vi "FPGA_HoppingScan_BoostedMultiRegion.vi"() -> ()   [LabVIEW 2024]
uses:
  <vilib>/Platform/TimedLoop/XDataNode/timing_clust.ctl
  <vilib>/Platform/TimedLoop/XDataNode/nitl_modes.ctl
  <vilib>/Platform/TimedLoop/XDataNode/wakeup.ctl
  <vilib>/rvi/FXPMathLib/FxpDiv/subVIs/nifxpmath_Div_SimConfig.ctl
  <vilib>/rvi/Emulation/niFpgaSctlEmulationGetInTimedLoop.vi
  <vilib>/rvi/Emulation/niFpgaProcessEmulError.vi
  <vilib>/rvi/eio/common/nirviEmuTemplateMethod_errors.vi
  <vilib>/rvi/Memory/Memory_Emulation/nirvimemoryFastEmulation.vi
  <vilib>/rvi/Memory/Memory_Emulation/nirvimemoryEmulation.vi
  <vilib>/rvi/Emulation/niFpgaEmulationIsFPGAContextNoSignature.vi
  <vilib>/rvi/DataTransferAndStorage/Container/Common/niFpgaContainerGetUniqueNameForEmu.vi
  <vilib>/rvi/errors/nirviReportUnexpectedCaseInternalError (U32).vi
  <vilib>/rvi/Emulation/niFpgaEmulationReportErrorSimple.vi
  <vilib>/rvi/Emulation/niFpgaGetClockAttributes.vi
  <vilib>/rvi/Emulation/niFpgaCriticalErrorInLSC.vi
  <vilib>/rvi/Memory/Memory_Emulation/niFpgaMemoryEmulationCacheClearOnFirstRun.vi
  <vilib>/rvi/Memory/Memory_Emulation/nirvimemoryEmulationManagerCache_MakeExclusive.vi
  <vilib>/rvi/Memory/Memory_Emulation/niFpgaMemoryEmulationValidateCache.vi
  <vilib>/rvi/Memory/Memory_Emulation/nirvimemoryEmulationManagerCache_InsertValue.vi
  <vilib>/Utility/error.llb/Clear Errors.vi
  <vilib>/rvi/Memory/Memory_Emulation/nirvimemoryEmulationManagerCache_ReleaseExclusive.vi
  <vilib>/rvi/Memory/Memory_Emulation/nirvimemoryEmulationManagerCache_GetValue.vi
  <vilib>/rvi/Memory/Memory_Emulation/nirvimemoryEmulationManagerCache_SetValue.vi
  <vilib>/rvi/FIFO/Fifo_Resource/nirvififoEmulationSetSize.vi
  <vilib>/rvi/FIFO/Fifo_Resource/nirviFifoEmulationQueueMgr.vi
  <instcachedir>/0/nirviFifoEmulationQueueMgr_E5CAEC123FF24DC58D834DCA3CDAA9B5.lvgen/nirviFifoEmulationQueueMgr_E5CAEC123FF24DC58D834DCA3CDAA9B5_001.vi
  <vilib>/rvi/errors/niFpgaSetErrorForExecOnDevCompSimple.vi
  <vilib>/rvi/eio/common/nirviEmuReportErrorAndStop.vi
  <vilib>/rvi/FIFO/Fifo_Resource/nirvififoEmulationCreateLock.vi
  <vilib>/rvi/FIFO/Fifo_Resource/nirvififoEmulationObtainLock.vi
  <vilib>/rvi/FIFO/Fifo_Resource/nirvififoEmulationReleaseLock.vi
  <vilib>/rvi/occurrence/nirviWaitOnOccurrenceBase.vi
  <vilib>/rvi/errors/nirviReportUnexpectedCaseInternalError.vi
  <vilib>/eio/utilities/niEioResolveVilibRelativePath.vi
  <vilib>/rvi/interface/RandomDataEmulation/niFpgaRandomDataHandleErrors.vi
  <vilib>/rvi/FXPMathLib/FxpDiv/simVIs/DllFxpDivTemp_sub.vi
  <vilib>/rvi/FIFO/Fifo_Resource/nirvififoEmulationDetermineInputValidOut.vi
  <vilib>/eio/EIONode/EIONode.xnode
  <vilib>/rvi/DataTransferAndStorage/Container/XNode/niFpgaContainer.xnode
  <vilib>/platform/TimedLoop/XDataNode/XDataNode.xnode
  <vilib>/rvi/DataTransferAndStorage/Register/Emulation/niFpgaRegisterEmulation.vi
  <vilib>/rvi/FIFO/Fifo_Resource/nirvififoEmulationGetNumberOfElementsToRead.vi
  <vilib>/rvi/FIFO/Fifo_Resource/nirvififoEmulationRead.vi
  <vilib>/rvi/interface/RandomDataEmulation/nirviRandomDataFpgaReadWriteTemplate.vi
  <vilib>/rvi/FXPMathLib/FxpSub/XNode/nifxpmath_Sub.xnode
  <vilib>/rvi/FXPMathLib/FxpAdd/XNode/nifxpmath_Add.xnode
  <vilib>/rvi/FXPMathLib/FxpMul/XNode/nifxpmath_Multiplier.xnode
  <vilib>/rvi/FXPMathLib/FxpDiv/XNode/nifxpmath_Div.xnode
  <vilib>/rvi/FIFO/Fifo_Resource/nirvififoEmulationWrite.vi
  <vilib>/rvi/FXPMathLib/sim/FxpSim.dll
  <vilib>/Platform/TimedLoop/XDataNode/XDNodeRunTimeDep.lvlib
panel:
  in  "Turning Distance":fxp<+/-,48,16>
  in  "LastScan":bool
  in  "InitScan":bool
  in  "DelayPoints":i32
  in  "Halting Threshold":fxp<+/-,48,16>
  out "point_scanned":u32
  in  "TotalPoints":u32
  in  "RetRate us":i32
  in  "AppRate_NF us":i32
  in  "AppRate_FF us":i32
  in  "Recording Threshold":fxp<+/-,48,16>
  in  "stop":bool
  out "TargetDone?":bool
  out "ScanFinished?":bool
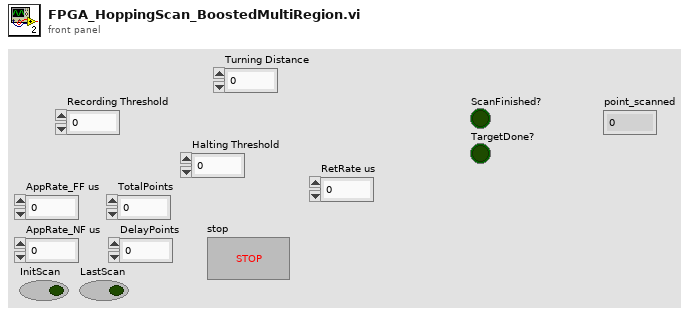
[diagram p1: front panel]
types:
  T1 = typedef "XDNodeRunTimeDep.lvlib/timing_clust.ctl" = cluster{"Expected End [f-1]":u64, "Actual End [f-1]":u64, "Finished Late? [f-1]":bool, "Expected End [i-1]":u64, "Actual End [i-1]":u64, "Finished Late? [i-1]":bool, "Expected Start [i]":u64, "Actual Start [i]":u64, "Expected Start [f]":u64, "Actual Start [f]":u64, "Source Name":string, "Structure Name":string, "Period":i64, "Deadline":i64, "Offset":i64, "Start":i64, "Priority":i32, "Timeout":i32, "Mode":T2, "Wakeup Reason":T3, "Error":errorcluster, "Source Type":string, "Secondary Source Type":string, "Global End Time":u64, "Global Start Time":u64, "Frame Duration":u64, "Iteration Duration":u64, "Assigned CPU":i32, "I/O Scan Engine Mode":u32}
  T2 = typedef "XDNodeRunTimeDep.lvlib/nitl_modes.ctl" = enum32{"No Change", "Process missed periods, maintain original phase", "Discard missed periods, maintain original phase", "Process missed periods, ignore original phase", "Discard missed periods, ignore original phase"}
  T3 = typedef "XDNodeRunTimeDep.lvlib/wakeup.ctl" = enum32{"Normal", "Aborted", "Asynchronous wakeup", "Timing source error", "Timed loop error", "Timeout"}
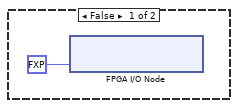
[diagram p2: hidden frame]
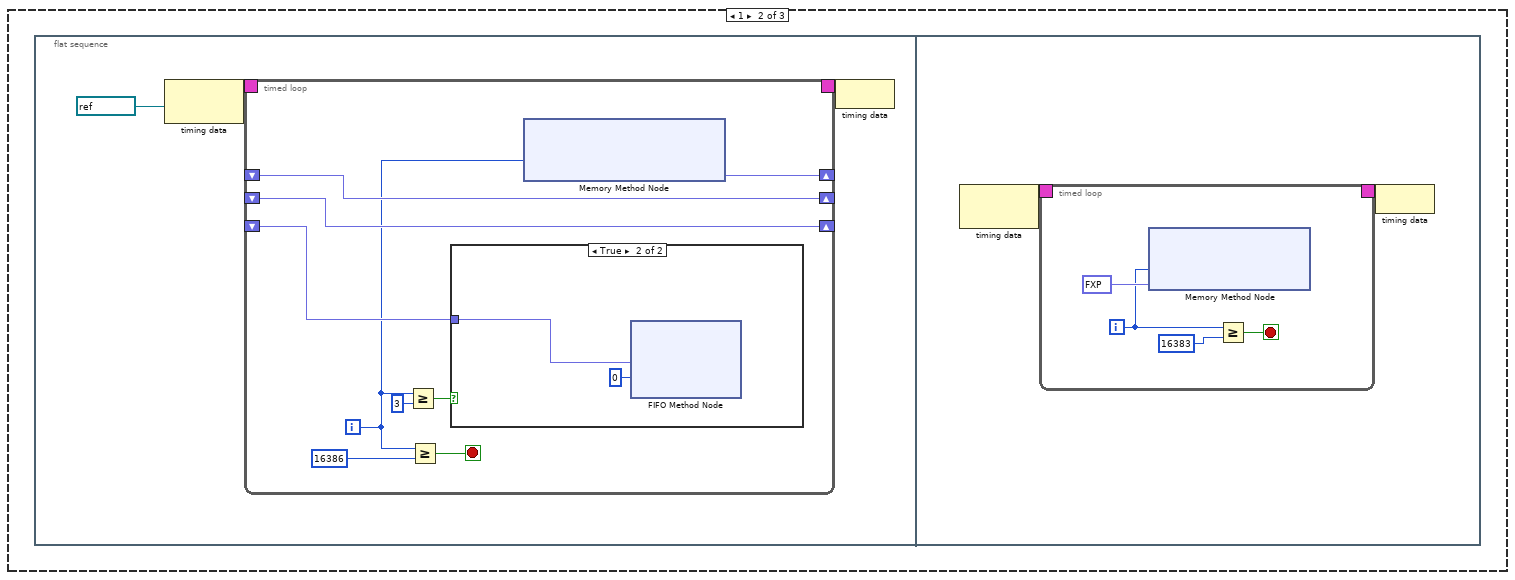
[diagram p5: hidden frame]
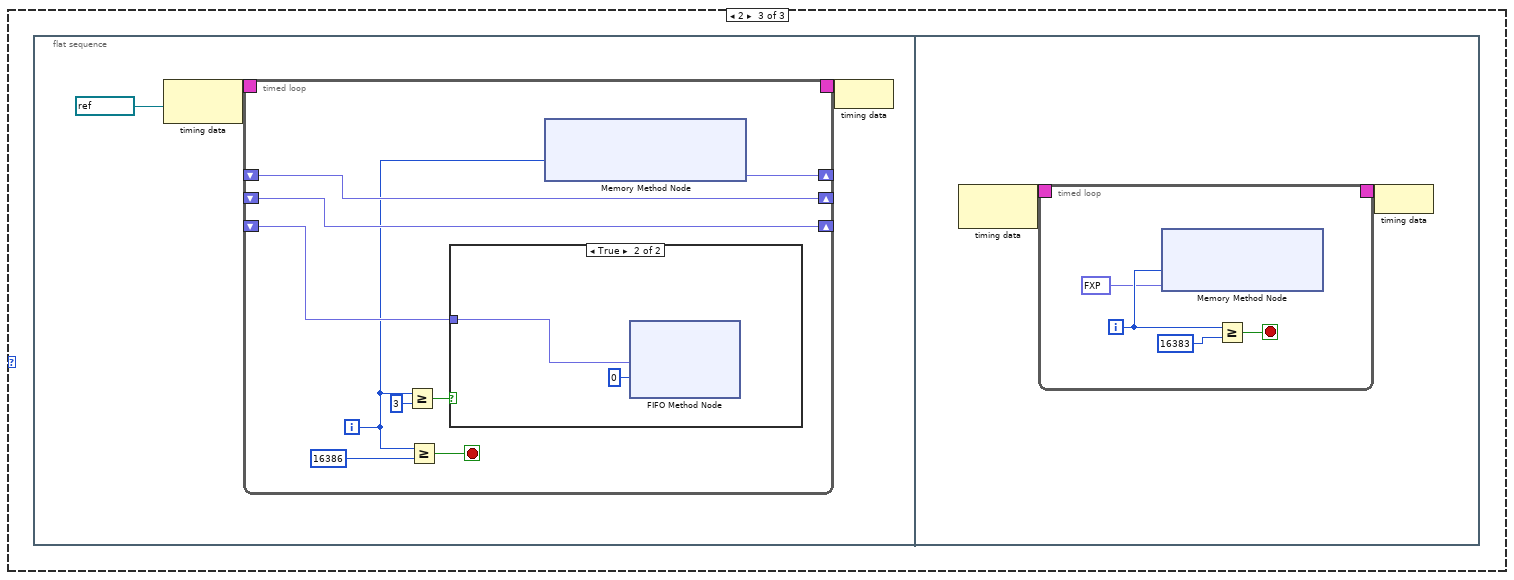
[diagram p7: hidden frame]
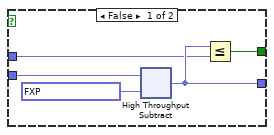
[diagram p14: hidden frame]
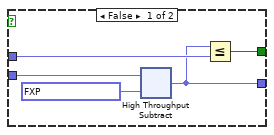
[diagram p15: hidden frame]
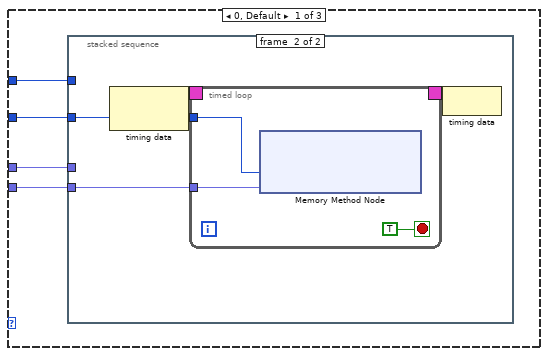
[diagram p18: hidden frame]
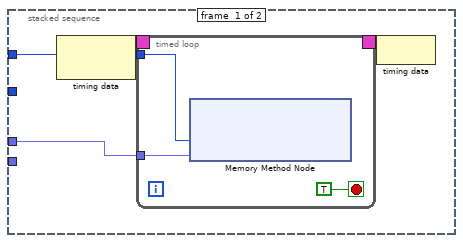
[diagram p19: hidden frame]
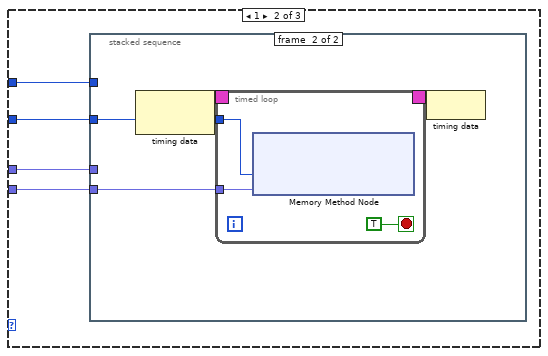
[diagram p20: hidden frame]
diagram:
  n1 = flat-sequence {
    tunnel: [w21] -> w1
    tunnel: w1 -> [w34]
    frame #0 {
      n2 = call "Wait18"("Count(mSec)"=u8 150) -> ()  [unwired: 1 out]
    }
    frame #1 {
      n3 = node-c288() -> (w5:T1)  [unwired: 1 in]
      n4 = timed-loop {
        timing: w5 -> [_]
        timing-out: [_] -> w4
        i -> [w14]
        stop <- w13 stop-if-true
        w16 = fxp<+/-,48,16> -100.0 ("Data")
        n5 = xnode ("Memory Method Node")("Address"=w14, "Data"=w16) -> ()  [unwired: 1 in, 1 out]
        n6 = xnode ("Memory Method Node")("Address"=w14, "Data"=w16) -> ()  [unwired: 1 in, 1 out]
        n7 = xnode ("Memory Method Node")("Address"=w14, "Data"=w16) -> ()  [unwired: 1 in, 1 out]
        n8 = Greater Or Equal?(x=w14, y=16383) -> (x >= y?=w13:bool)
      }
      n9 = case shown="True" "InitScan" {
        frame False {
          n10 = xnode "FPGA I/O Node"("Connector0/AO2"=fxp<+/-,20,5> 0.0 ("Connector0/AO0")) -> ()  [unwired: 1 in, 1 out]
        }
        frame True {
          w10 = fxp<+/-,20,5> 0.0 ("Connector0/AO0")
          n11 = for {
            N: 6 -> [_]
            i -> [w12]
            n12 = xnode ("Memory Method Node")("Address"=w12, "Data"=fxp<+/-,48,16> 0.0) -> ()  [unwired: 1 in, 1 out]
          }
          n13 = xnode "FPGA I/O Node"("Connector0/AO0"=w10, "Connector0/AO1"=w10, "Connector0/AO2"=w10) -> ()  [unwired: 3 in, 3 out]
        }
      }
      n14 = node-c288(w4) -> ()
      "ScanFinished?" <- FALSE
      "TargetDone?" <- FALSE
    }
    frame #2 {
      n15 = Generate Occurrence() -> (w21:refnum<k4>)
      n16 = call "Wait"("Count(mSec)"=u8 50) -> ()  [unwired: 1 out]
    }
    frame #3 {
      n17 = while {
        tunnel: w34 -> [w151]
        stop <- w153 stop-if-true
        n18 = xnode ("Register Read")() -> ("Data"=w154:bool)  [unwired: 1 in, 1 out]
        n19 = xnode ("FIFO Method Node")() -> ("Number of Elements to Read"=w157:u32)  [unwired: 1 in, 1 out]
        n20 = local read "ScanFinished?"() -> (w152:bool)
        n21 = Or(x=w154, y=w152) -> (x .or. y?=w153:bool)
        n22 = Greater Or Equal?(x=w157, y=u32 6) -> (x >= y?=w155:bool)
        n23 = case shown="True" w155 {
          tunnel: w151 -> [_ w158]
          frame False {
          }
          frame True {
            n24 = First Call?() -> (First Call?: T/F=w159:bool)
            n25 = case shown="True" w159 {
              tunnel: w158 -> [_ w160]
              frame False {
              }
              frame True {
                n26 = flat-sequence {
                  tunnel: [w163] -> w161
                  tunnel: w160 -> [w163]
                  tunnel: w161 -> [w164]
                  frame #0 {
                    n27 = call "Wait3"("Count(mSec)"=u8 4) -> ()  [unwired: 1 out]
                  }
                  frame #1 {
                    n28 = Set Occurrence(w164) -> ()
                  }
                }
              }
            }
          }
        }
      }
      n29 = while {
        tunnel: w34 -> [w136]
        stop <- w133 stop-if-true
        n30 = flat-sequence {
          tunnel: ["stop"] -> w138
          tunnel: w136 -> [w140]
          tunnel: [w140] -> w134
          tunnel: w138 -> [w143]
          tunnel: [w143] -> w137
          tunnel: [w142] -> w135
          tunnel: w134 -> [w142]
          tunnel: w137 -> [w147]
          tunnel: w135 -> [w146]
          tunnel: [w145] -> w133
          frame #0 {
            n31 = case shown="True" "stop" {
              tunnel: "stop" -> [_ w141]
              frame False {
              }
              frame True {
                n32 = xnode ("Register Write")("Data"=w141) -> ()  [unwired: 1 in, 1 out]
              }
            }
          }
          frame #1 {
            n33 = call "Wait2"("Count(uSec)"=u8 200) -> ()  [unwired: 1 out]
          }
          frame #2 {
            n34 = xnode ("Register Read")() -> ("Data"=w148:bool)  [unwired: 1 in, 1 out]
            n35 = local read "ScanFinished?"() -> (w149:bool)
            n36 = Compound Arithmetic op=OR(w149, w148, w147) -> (w145:bool)
            n37 = case shown="True" w145 {
              tunnel: w146 -> [_ w150]
              frame False {
              }
              frame True {
                n38 = Set Occurrence(w150) -> ()
              }
            }
          }
        }
      }
      n39 = flat-sequence {
        tunnel: w34 -> [w165]
        tunnel: [fxp<+/-,48,16> 0.0 ("Threshold")] -> w33
        tunnel: [w167] -> w31
        tunnel: [u8 0] -> w28
        tunnel: w33 -> [w170]
        tunnel: [w171] -> w32
        tunnel: w31 -> [w171]
        tunnel: [w170] -> w30
        tunnel: [w169] -> w29
        tunnel: w28 -> [w169]
        tunnel: w32 -> [w176]
        tunnel: w30 -> [w175]
        tunnel: w29 -> [w174]
        tunnel: [w173] -> w27
        tunnel: w27 -> [w1243]
        tunnel: [w1242] -> w26
        tunnel: [w1241] -> w24
        tunnel: w26 -> [w1255]
        tunnel: [w1255] -> w25
        tunnel: w24 -> [w1254]
        tunnel: [w1254] -> w23
        tunnel: w25 -> [w1260]
        tunnel: w23 -> [w1259]
        frame #0 {
          n40 = Wait on Occurrence(2:w165) -> ()  [unwired: 2 in, 1 out]
        }
        frame #1 {
          # "z piezo voltage"
          # "Swapchain indicator"
          n41 = xnode ("Register Read")() -> ("Data"=w167:bool)  [unwired: 1 in, 1 out]
        }
        frame #2 {
          n42 = call "Wait4"("Count(mSec)"=u8 4) -> ()  [unwired: 1 out]
        }
        frame #3 {
          n43 = case shown="False" w176 {
            tunnel: w175 -> [w179 w1239]
            tunnel: w174 -> [w178 _]
            tunnel: [w177 w1239] -> w173
            frame False {
              n44 = while {
                shift-right: [w186] -> w177
                shift-left: w179 -> [w213]
                shift-right: [w185] -> _
                shift-left: w178 -> [w196]
                stop <- w184 stop-if-true
                n45 = flat-sequence {
                  tunnel: w213 -> [w215]
                  tunnel: [w217] -> w212
                  tunnel: [w216] -> w208
                  tunnel: [w215] -> w200
                  tunnel: w196 -> [w214]
                  tunnel: [w214] -> w195
                  tunnel: w212 -> [w225]
                  tunnel: [w225] -> w211
                  tunnel: w208 -> [w224]
                  tunnel: [w224] -> w207
                  tunnel: w200 -> [w223]
                  tunnel: [w223] -> w199
                  tunnel: w195 -> [w222]
                  tunnel: [w222] -> w194
                  tunnel: w211 -> [w252]
                  tunnel: [w252] -> w210
                  tunnel: [w245] -> w209
                  tunnel: w207 -> [w251]
                  tunnel: [w251] -> w206
                  tunnel: [w246] -> w205
                  tunnel: [w249] -> w204
                  tunnel: [w248] -> w203
                  tunnel: [w247] -> w202
                  tunnel: w199 -> [w244]
                  tunnel: w194 -> [w250]
                  tunnel: [w250] -> w193
                  tunnel: [w241] -> w183
                  tunnel: [w243] -> w180
                  tunnel: [w289] -> w201
                  tunnel: [w288] -> w198
                  tunnel: [w287] -> w191
                  tunnel: [w286] -> w190
                  tunnel: [w285] -> w189
                  tunnel: [w284] -> w182
                  tunnel: w180 -> [w288]
                  tunnel: w183 -> [w284]
                  tunnel: w193 -> [w287]
                  tunnel: w202 -> [w285]
                  tunnel: w203 -> [w286]
                  tunnel: w204 -> [w289]
                  tunnel: w205 -> [w291]
                  tunnel: w206 -> [w290]
                  tunnel: w209 -> [w281]
                  tunnel: w210 -> [w280]
                  tunnel: w201 -> [w335]
                  tunnel: w198 -> [w334]
                  tunnel: [w334] -> w197
                  tunnel: [w333] -> w192
                  tunnel: w191 -> [w333]
                  tunnel: w190 -> [w332]
                  tunnel: w189 -> [w331]
                  tunnel: [w332] -> w188
                  tunnel: [w331] -> w187
                  tunnel: w182 -> [w330]
                  tunnel: [w330] -> w181
                  tunnel: w197 -> [w350]
                  tunnel: w192 -> [w349]
                  tunnel: w188 -> [w348]
                  tunnel: w187 -> [w347]
                  tunnel: [w346] -> w185
                  tunnel: [w345] -> w186
                  tunnel: [w344] -> w184
                  tunnel: w181 -> [w340]
                  frame #0 {
                    # "Data from target to host:\n0, 1: X, Y piezo voltage\n2, 3: X, Y piezo idx\n4: Z piezo probing voltage\n5: Z piezo final voltage\n6: baseline current\n7: circular buffer pointer idx\n(8-8107): Z voltage\n(8108-16207): current\n(8107-16206): current"
                    # "Data from host to target:\n0, 1: X, Y piezo voltage\n2, 3: X, Y piezo idx\n4: distance (piezo voltage) to the last point\n5: retract height, \nall negative cases won't trigger approach of z piezo\nif -20, keep z and move xy\nif -30, full retract for z and move xy"
                    n46 = for {
                      N: 2 -> [_]
                      shift-right: [w221] -> w216
                      shift-left: _ -> [w219]
                      shift-right: [w219] -> w217
                      shift-left: _ -> [_]
                      i -> [w220]
                      n47 = xnode ("Memory Method Node")("Address"=w220) -> ("Data"=w221:fxp<+/-,48,16>)  [unwired: 1 in, 1 out]
                    }
                  }
                  frame #1 {
                    # "y"
                    # "x"
                    n48 = while {
                      shift-right: [w229] -> _
                      shift-left: i16 0 -> [w228]
                      stop <- w230 stop-if-true
                      n49 = xnode ("FIFO Method Node")("Timeout"=8192) -> ("Element"=w227:fxp<+/-,48,16>, "Timed Out?"=w234:bool)  [unwired: 1 in, 1 out]
                      n50 = Increment(x=w228) -> (x+1=w237:i16)
                      n51 = xnode ("Register Read")() -> ("Data"=w231:bool)  [unwired: 1 in, 1 out]
                      n52 = Select(t=w228, s=w234, f=w237) -> (s? t:f=w229:i16)
                      n53 = Not(x=w234) -> (.not. x?=w233:bool)
                      n54 = Equal?(x=w228, y=i16 5) -> (x = y?=w235:bool)
                      n55 = And(x=w235, y=w233) -> (x .and. y?=w232:bool)
                      n56 = xnode ("Memory Method Node")("Address"=w228, "Data"=w227) -> ()  [unwired: 1 in, 1 out]
                      n57 = Or(x=w232, y=w231) -> (x .or. y?=w230:bool)
                    }
                  }
                  frame #2 {
                    # "0"
                    # "5"
                    n58 = for {
                      N: 6 -> [_]
                      shift-right: [w278] -> w241
                      shift-left: _ -> [w277]
                      shift-right: [w277] -> w249
                      shift-left: _ -> [w276]
                      shift-right: [w276] -> w248
                      shift-left: _ -> [w275]
                      shift-right: [w275] -> w247
                      shift-left: _ -> [w274]
                      shift-right: [w274] -> w246
                      shift-left: _ -> [w273]
                      shift-right: [w273] -> w245
                      shift-left: _ -> [_]
                      i -> [w279]
                      n59 = xnode ("Memory Method Node")("Address"=w279) -> ("Data"=w278:fxp<+/-,48,16>)  [unwired: 1 in, 1 out]
                    }
                    n60 = Equal?(x=w241, y=fxp<+/-,48,16> -30.0) -> (x = y?=w240:bool)
                    n61 = case shown="True" w240 {
                      tunnel: w244 -> [w254 w258]
                      tunnel: [w254 w257] -> w243
                      tunnel: fxp<+/-,48,16> 0.0048828125 ("y") -> [_ w256]
                      frame False {
                      }
                      frame True {
                        n62 = flat-sequence {
                          tunnel: w258 -> [w261]
                          tunnel: w256 -> [w259]
                          tunnel: [w260] -> w255
                          tunnel: [w272] -> w257
                          tunnel: w255 -> [w272]
                          frame #0 {
                            n63 = while {
                              shift-right: [w265] -> w260
                              shift-left: w261 -> [w270]
                              tunnel: w259 -> [w264]
                              stop <- w266 stop-if-true
                              w267 = fxp<+/-,48,16> 0.0 ("y")
                              n64 = xnode "High Throughput Subtract"("x"=w270, "y"=w264) -> ("x-y"=w268:fxp<+/-,48,16>)
                              n65 = xnode ("Register Read")() -> ("Data"=w269:bool)  [unwired: 1 in, 1 out]
                              n66 = Less Or Equal?(x=w268, y=w267) -> (x <= y?=w262:bool)
                              n67 = Select(t=w267, s=w262, f=w268) -> (s? t:f=w265:fxp<+/-,48,16>)
                              n68 = local read "RetRate us"() -> (w263:i32)
                              n69 = xnode "FPGA I/O Node"("Connector0/AO2"=w265) -> ()  [unwired: 1 in, 1 out]
                              n70 = Compound Arithmetic op=OR(w262, w269) -> (w266:bool)
                              n71 = call "Wait10"("Count(uSec)"=w263) -> ()  [unwired: 1 out]
                            }
                          }
                          frame #1 {
                            n72 = call "Wait17"("Count(mSec)"=u16 2 ("Count(uSec)")) -> ()  [unwired: 1 out]
                          }
                        }
                      }
                    }
                  }
                  frame #3 {
                    n73 = xnode "High Throughput Subtract"("x"=w290, "y"=w291) -> ("x-y"=w293:fxp<+/-,48,16>)
                    n74 = xnode "High Throughput Subtract"("x"=w280, "y"=w281) -> ("x-y"=w283:fxp<+/-,48,16>)
                    n75 = Less Or Equal To 0?(x=w293) -> (x <= 0?=w292:bool)
                    n76 = Less Or Equal To 0?(x=w283) -> (x <= 0?=w282:bool)
                    n77 = while {
                      tunnel: w292 -> [w319]
                      tunnel: w291 -> [w318]
                      shift-right: [w312] -> _
                      shift-left: w290 -> [w314]
                      stop <- w315 stop-if-true
                      n78 = case shown="True" w319 {
                        tunnel: w318 -> [w321 w326]
                        tunnel: w314 -> [w323 w329]
                        tunnel: [w322 w327] -> w313
                        tunnel: [w320 w325] -> w312
                        frame False {
                          n79 = xnode "High Throughput Subtract"("x"=w323, "y"=fxp<+/-,48,16> 0.00030517578125) -> ("x-y"=w320:fxp<+/-,48,16>)
                          n80 = Less Or Equal?(x=w320, y=w321) -> (x <= y?=w322:bool)
                        }
                        frame True {
                          n81 = xnode ("High Throughput Add")("x"=w329, "y"=fxp<+/-,48,16> 0.00030517578125) -> ("x+y"=w325:fxp<+/-,48,16>)
                          n82 = Greater Or Equal?(x=w325, y=w326) -> (x >= y?=w327:bool)
                        }
                      }
                      n83 = call "Wait6"("Count(uSec)"=u32 70) -> ()  [unwired: 1 out]
                      n84 = xnode ("Register Read")() -> ("Data"=w316:bool)  [unwired: 1 in, 1 out]
                      n85 = xnode "FPGA I/O Node"("Connector0/AO1"=w312) -> ()  [unwired: 1 in, 1 out]
                      n86 = Or(x=w313, y=w316) -> (x .or. y?=w315:bool)
                    }
                    n87 = while {
                      tunnel: w282 -> [w301]
                      tunnel: w281 -> [w300]
                      shift-right: [w294] -> _
                      shift-left: w280 -> [w296]
                      stop <- w297 stop-if-true
                      n88 = case shown="True" w301 {
                        tunnel: w300 -> [w302 w307]
                        tunnel: w296 -> [w305 w311]
                        tunnel: [w304 w309] -> w295
                        tunnel: [w303 w308] -> w294
                        frame False {
                          n89 = xnode "High Throughput Subtract"("x"=w305, "y"=fxp<+/-,48,16> 0.00030517578125) -> ("x-y"=w303:fxp<+/-,48,16>)
                          n90 = Less Or Equal?(x=w303, y=w302) -> (x <= y?=w304:bool)
                        }
                        frame True {
                          n91 = xnode ("High Throughput Add")("x"=w311, "y"=fxp<+/-,48,16> 0.00030517578125) -> ("x+y"=w308:fxp<+/-,48,16>)
                          n92 = Greater Or Equal?(x=w308, y=w307) -> (x >= y?=w309:bool)
                        }
                      }
                      n93 = call "Wait5"("Count(uSec)"=u32 70) -> ()  [unwired: 1 out]
                      n94 = xnode ("Register Read")() -> ("Data"=w298:bool)  [unwired: 1 in, 1 out]
                      n95 = xnode "FPGA I/O Node"("Connector0/AO0"=w294) -> ()  [unwired: 1 in, 1 out]
                      n96 = Or(x=w295, y=w298) -> (x .or. y?=w297:bool)
                    }
                  }
                  frame #4 {
                    n97 = xnode ("High Throughput Multiply")("x"=w335, "y"=fxp<+/-,48,16> 1600.0) -> ("x*y"=w337:fxp<+/-,52,20>)
                    n98 = To Unsigned Long Integer(number=w337) -> (unsigned 32bit integer=w338:u32)
                    n99 = call "Wait7"("Count(uSec)"=w338) -> ()  [unwired: 1 out]
                  }
                  frame #5 {
                    # "Y, X idx"
                    n100 = xnode ("Register Read")() -> ("Data"=w343:bool)  [unwired: 1 in, 1 out]
                    n101 = Less Or Equal?(x=w340, y=fxp<+/-,48,16> -20.0) -> (x <= y?=w341:bool)
                    n102 = Or(x=w341, y=w343) -> (x .or. y?=w342:bool)
                    n103 = case shown="False" w342 {
                      tunnel: w350 -> [w397 w1238]
                      tunnel: w349 -> [w396 w1237]
                      tunnel: w348 -> [w392 _]
                      tunnel: w347 -> [w391 _]
                      tunnel: [w389 w1238] -> w345
                      tunnel: [w390 w1237] -> w346
                      tunnel: [w388 w1234] -> w344
                      tunnel: w341 -> [_ w1236]
                      tunnel: w340 -> [w384 _]
                      frame False {
                        n104 = flat-sequence {
                          tunnel: [w399] -> w382
                          tunnel: [w404] -> w381
                          tunnel: [w403] -> w380
                          tunnel: w397 -> [w402]
                          tunnel: [w402] -> w379
                          tunnel: w396 -> [w401]
                          tunnel: [w401] -> w378
                          tunnel: [0] -> w377
                          tunnel: [w399] -> w376
                          tunnel: w382 -> [w442]
                          tunnel: [w441] -> w375
                          tunnel: w381 -> [w443]
                          tunnel: w380 -> [w449]
                          tunnel: [w449] -> w374
                          tunnel: w379 -> [w445]
                          tunnel: [w444] -> w373
                          tunnel: w378 -> [w448]
                          tunnel: [w448] -> w372
                          tunnel: w377 -> [w447]
                          tunnel: [w447] -> w371
                          tunnel: w376 -> [w446]
                          tunnel: [w446] -> w370
                          tunnel: [w440] -> w369
                          tunnel: w375 -> [w533]
                          tunnel: [w533] -> w364
                          tunnel: w374 -> [w532]
                          tunnel: [w532] -> w362
                          tunnel: w373 -> [w524]
                          tunnel: [w522] -> w360
                          tunnel: w372 -> [w531]
                          tunnel: [w531] -> w358
                          tunnel: w371 -> [w530]
                          tunnel: [w530] -> w356
                          tunnel: w370 -> [w529]
                          tunnel: [w529] -> w354
                          tunnel: w369 -> [w521]
                          tunnel: [w521] -> w352
                          tunnel: w364 -> [w558]
                          tunnel: [w558] -> w363
                          tunnel: w362 -> [w557]
                          tunnel: [w557] -> w361
                          tunnel: w360 -> [w556]
                          tunnel: [w556] -> w359
                          tunnel: w358 -> [w555]
                          tunnel: [w555] -> w357
                          tunnel: w356 -> [w554]
                          tunnel: [w554] -> w355
                          tunnel: w354 -> [w553]
                          tunnel: [w553] -> w353
                          tunnel: w352 -> [w552]
                          tunnel: [w552] -> w351
                          tunnel: w363 -> [w568]
                          tunnel: w361 -> [w567]
                          tunnel: w359 -> [w566]
                          tunnel: w357 -> [w565]
                          tunnel: w355 -> [w560]
                          tunnel: [w564] -> w395
                          tunnel: [w563] -> w394
                          tunnel: [w562] -> w393
                          tunnel: w353 -> [w561]
                          tunnel: [w561] -> w383
                          tunnel: w351 -> [w559]
                          tunnel: [w559] -> w368
                          tunnel: w395 -> [w851]
                          tunnel: w394 -> [w853]
                          tunnel: w393 -> [w854]
                          tunnel: w392 -> [w856]
                          tunnel: w391 -> [w855]
                          tunnel: [w852] -> w387
                          tunnel: [w851] -> w386
                          tunnel: [w848] -> w385
                          tunnel: w383 -> [w847]
                          tunnel: w368 -> [w846]
                          tunnel: w387 -> [w1211]
                          tunnel: w386 -> [w1207]
                          tunnel: w385 -> [w1210]
                          tunnel: w384 -> [w1208]
                          tunnel: [w1211] -> w367
                          tunnel: [w1209] -> w366
                          tunnel: [w1210] -> w365
                          tunnel: [w1230] -> w388
                          tunnel: [w1231] -> w389
                          tunnel: [w1232] -> w390
                          tunnel: w367 -> [w1232]
                          tunnel: w366 -> [w1231]
                          tunnel: w365 -> [w1230]
                          frame #0 {
                            n105 = for {
                              N: 32 -> [_]
                              shift-right: [w437] -> w407
                              shift-left: fxp<+/-,48,16> 0.0 -> [w438]
                              n106 = xnode "FPGA I/O Node"() -> ("Connector0/AI3"=w439:fxp<+/-,27,5>)  [unwired: 1 in, 1 out]
                              n107 = xnode ("High Throughput Add")("x"=w439, "y"=w438) -> ("x+y"=w437:fxp<+/-,48,16>)
                            }
                            n108 = local read "Halting Threshold"() -> (w398:fxp<+/-,48,16>)
                            n109 = local read "Recording Threshold"() -> (w405:fxp<+/-,48,16>)
                            n110 = xnode "High Throughput Divide"("x"=w407, "y"=fxp<+/-,48,16> 32.0) -> ("x/y"=w399:fxp<+/-,48,16>)
                            n111 = xnode ("High Throughput Multiply")("x"=w399, "y"=w405) -> ("x*y"=w404:fxp<+/-,48,16>)
                            n112 = xnode ("High Throughput Multiply")("x"=w399, "y"=w398) -> ("x*y"=w403:fxp<+/-,48,16>)
                          }
                          frame #1 {
                            n113 = while {
                              shift-right: [w451] -> w444
                              shift-left: w445 -> [w457]
                              tunnel: w443 -> [w462]
                              tunnel: w442 -> [w461]
                              tunnel: [w460] -> w441
                              tunnel: [w450] -> w440
                              stop <- w454 stop-if-true
                              n114 = flat-sequence {
                                tunnel: w462 -> [w475]
                                tunnel: w461 -> [w477]
                                tunnel: [w477] -> w459
                                tunnel: w457 -> [w464]
                                tunnel: [w466] -> w455
                                tunnel: [w463] -> w453
                                tunnel: w459 -> [w516]
                                tunnel: [w516] -> w458
                                tunnel: [w515] -> w456
                                tunnel: w455 -> [w515]
                                tunnel: w453 -> [w514]
                                tunnel: [w514] -> w452
                                tunnel: [w520] -> w460
                                tunnel: w458 -> [w520]
                                tunnel: w456 -> [w519]
                                tunnel: [w519] -> w454
                                tunnel: w452 -> [w517]
                                tunnel: [w517] -> w451
                                tunnel: [w517] -> w450
                                frame #0 {
                                w483 = 16
                                n115 = for {
                                N: w483 -> [_]
                                shift-right: [w511] -> w481
                                shift-left: fxp<+/-,48,16> 0.0 ("y") -> [w513]
                                n116 = xnode "FPGA I/O Node"() -> ("Connector0/AI3"=w512:fxp<+/-,27,5>)  [unwired: 2 in, 3 out]
                                n117 = xnode ("High Throughput Add")("x"=w513, "y"=w512) -> ("x+y"=w511:fxp<+/-,48,16>)
                                }
                                n118 = To Fixed-Point(number=w483) -> (fixed-point=w482:fxp<+/-,48,16>)  [unwired: 1 in]
                                n119 = xnode ("High Throughput Add")("x"=w464, "y"=fxp<+/-,48,16> 0.00030517578125) -> ("x+y"=w465:fxp<+/-,48,16>)
                                n120 = xnode ("Register Read")() -> ("Data"=w467:bool)  [unwired: 1 in, 1 out]
                                n121 = Greater?(x=w465, y=fxp<+/-,48,16> 9.75) -> (0:w473:bool)
                                n122 = Less?(x=w465, y=fxp<+/-,48,16> -0.125) -> (x < y?=w474:bool)
                                n123 = Or(x=w474, y=w473) -> (x .or. y?=w468:bool)
                                n124 = xnode "High Throughput Divide"("x"=w481, "y"=w482) -> ("x/y"=w478:fxp<+/-,48,16>)
                                n125 = xnode "High Throughput Subtract"("x"=w477, "y"=w478) -> ("x-y"=w479:fxp<+/-,48,16>)
                                n126 = Absolute Value(x=w479) -> (abs(x)=w476:fxp<+,48,16>)
                                n127 = Greater Or Equal?(x=w476, y=w475) -> (x >= y?=w469:bool)
                                n128 = Compound Arithmetic op=OR(w469, w467, w468) -> (w466:bool)
                                n129 = Select(t=w464, s=w466, f=w465) -> (s? t:f=w463:fxp<+/-,48,16>)
                                }
                                frame #1 {
                                n130 = xnode "FPGA I/O Node"("Connector0/AO2"=w514) -> ()  [unwired: 1 in, 1 out]
                                }
                                frame #2 {
                                n131 = local read "AppRate_FF us"() -> (w518:i32)
                                n132 = call "Wait19"("Count(uSec)"=w518) -> ()  [unwired: 1 out]
                                }
                              }
                            }
                          }
                          frame #2 {
                            n133 = xnode ("Register Read")() -> ("Data"=w528:bool)  [unwired: 1 in, 1 out]
                            n134 = local read "Turning Distance"() -> (w523:fxp<+/-,48,16>)
                            n135 = Less Or Equal To 0?(x=w524) -> (x <= 0?=w527:bool)
                            n136 = Or(x=w528, y=w527) -> (x .or. y?=w526:bool)
                            n137 = case shown="False" w526 {
                              tunnel: w524 -> [w536 w550]
                              tunnel: [w538 w550] -> w522
                              tunnel: fxp<+/-,48,16> 0.00030517578125 ("y") -> [w537 _]
                              tunnel: w523 -> [w534 _]
                              frame False {
                                n138 = xnode "High Throughput Subtract"("x"=w536, "y"=w534) -> ("x-y"=w535:fxp<+/-,48,16>)
                                n139 = while {
                                shift-right: [w543] -> w538
                                shift-left: w536 -> [w549]
                                tunnel: w537 -> [w542]
                                tunnel: w535 -> [w541]
                                stop <- w544 stop-if-true
                                n140 = xnode "High Throughput Subtract"("x"=w549, "y"=w542) -> ("x-y"=w545:fxp<+/-,48,16>)
                                n141 = xnode ("Register Read")() -> ("Data"=w548:bool)  [unwired: 1 in, 1 out]
                                n142 = Less Or Equal To 0?(x=w545) -> (x <= 0?=w546:bool)
                                n143 = Less Or Equal?(x=w545, y=w541) -> (x <= y?=w547:bool)
                                n144 = Select(t=fxp<+/-,48,16> 0.0, s=w546, f=w545) -> (s? t:f=w543:fxp<+/-,48,16>)
                                n145 = local read "RetRate us"() -> (w539:i32)
                                n146 = xnode "FPGA I/O Node"("Connector0/AO2"=w543) -> ()  [unwired: 1 in, 1 out]
                                n147 = Compound Arithmetic op=OR(w546, w547, w548) -> (w544:bool)
                                n148 = call "Wait20"("Count(uSec)"=w539) -> ()  [unwired: 1 out]
                                }
                              }
                              frame True {
                              }
                            }
                          }
                          frame #3 {
                            n149 = call "Wait22"("Count(mSec)"=u8 5) -> ()  [unwired: 1 out]
                          }
                          frame #4 {
                            n150 = while {
                              tunnel: w568 -> [w614]
                              tunnel: w567 -> [w613]
                              shift-right: [w597] -> w564
                              shift-left: w566 -> [w612]
                              shift-right: [w596] -> w563
                              shift-left: w565 -> [w611]
                              shift-right: [w582] -> _
                              shift-left: w560 -> [w604]
                              tunnel: [w590] -> w562
                              shift-right: [w569] -> _
                              shift-left: w560 -> [w573]
                              stop <- w593 stop-if-true
                              n151 = flat-sequence {
                                tunnel: w604 -> [w617]
                                tunnel: w611 -> [w618]
                                tunnel: w612 -> [w619]
                                tunnel: w613 -> [w620]
                                tunnel: w614 -> [w621]
                                tunnel: [w621] -> w589
                                tunnel: [w620] -> w588
                                tunnel: [w619] -> w587
                                tunnel: [w618] -> w586
                                tunnel: [w617] -> w585
                                tunnel: [w616] -> w584
                                tunnel: [w615] -> w574
                                tunnel: w573 -> [w615]
                                tunnel: [w655] -> w610
                                tunnel: [w643] -> w608
                                tunnel: [w640] -> w607
                                tunnel: [w654] -> w603
                                tunnel: [w653] -> w601
                                tunnel: [w652] -> w598
                                tunnel: [w635] -> w595
                                tunnel: [w645] -> w591
                                tunnel: w589 -> [w659]
                                tunnel: w588 -> [w636]
                                tunnel: w587 -> [w656]
                                tunnel: w586 -> [w653]
                                tunnel: w585 -> [w654]
                                tunnel: w584 -> [w639]
                                tunnel: [w639] -> w583
                                tunnel: w574 -> [w627]
                                tunnel: [w628] -> w571
                                tunnel: w610 -> [w729]
                                tunnel: [w729] -> w609
                                tunnel: w608 -> [w728]
                                tunnel: w607 -> [w727]
                                tunnel: [w728] -> w606
                                tunnel: [w727] -> w605
                                tunnel: w603 -> [w726]
                                tunnel: [w726] -> w602
                                tunnel: w601 -> [w725]
                                tunnel: [w725] -> w600
                                tunnel: [w724] -> w599
                                tunnel: w598 -> [w724]
                                tunnel: w595 -> [w723]
                                tunnel: [w723] -> w594
                                tunnel: [w722] -> w592
                                tunnel: w591 -> [w722]
                                tunnel: w583 -> [w721]
                                tunnel: [w721] -> w576
                                tunnel: [w720] -> w572
                                tunnel: w571 -> [w720]
                                tunnel: w609 -> [w741]
                                tunnel: w606 -> [w743]
                                tunnel: w605 -> [w742]
                                tunnel: w602 -> [w732]
                                tunnel: w600 -> [w740]
                                tunnel: w599 -> [w734]
                                tunnel: w594 -> [w739]
                                tunnel: w592 -> [w738]
                                tunnel: [w744] -> w581
                                tunnel: [w741] -> w580
                                tunnel: [w740] -> w579
                                tunnel: [w739] -> w578
                                tunnel: [w738] -> w577
                                tunnel: w576 -> [w736]
                                tunnel: [w736] -> w575
                                tunnel: w572 -> [w735]
                                tunnel: [w735] -> w570
                                tunnel: [w841] -> w590
                                tunnel: [w842] -> w593
                                tunnel: [w843] -> w596
                                tunnel: [w844] -> w597
                                tunnel: [w845] -> w582
                                tunnel: w581 -> [w845]
                                tunnel: w580 -> [w844]
                                tunnel: w579 -> [w843]
                                tunnel: w578 -> [w842]
                                tunnel: w577 -> [w841]
                                tunnel: w575 -> [w839]
                                tunnel: [w833] -> w569
                                tunnel: w570 -> [w833]
                                frame #0 {
                                n152 = call "Tick Count"() -> ("Tick Count(uSec)"=w616:u32)
                                }
                                frame #1 {
                                w625 = 16
                                w657 = fxp<+/-,48,16> 0.0 ("y")
                                # "brake zone"
                                # "recording zone"
                                n153 = for {
                                N: w625 -> [_]
                                shift-right: [w717] -> w644
                                shift-left: w657 -> [w718]
                                shift-right: [w714] -> w642
                                shift-left: w657 -> [w716]
                                n154 = xnode "FPGA I/O Node"() -> ("Connector0/AI2"=w719:fxp<+/-,27,5>, "Connector0/AI3"=w715:fxp<+/-,27,5>)  [unwired: 2 in, 2 out]
                                n155 = xnode ("High Throughput Add")("x"=w716, "y"=w715) -> ("x+y"=w714:fxp<+/-,48,16>)
                                n156 = xnode ("High Throughput Add")("x"=w719, "y"=w718) -> ("x+y"=w717:fxp<+/-,48,16>)
                                }
                                n157 = To Fixed-Point(number=w625) -> (fixed-point=w641:fxp<+/-,48,16>)  [unwired: 1 in]
                                n158 = local read "DelayPoints"() -> (w624:i32)
                                n159 = Not Equal To 0?(x=w627) -> (x != 0?=w626:bool)
                                n160 = Add(x=w627, y=1) -> (x+y=w629:i32)
                                n161 = Greater Or Equal?(x=w627, y=w624) -> (x >= y?=w631:bool)
                                n162 = Select(t=0, s=w631, f=w629) -> (s? t:f=w628:i32)
                                n163 = Select(t=fxp<+/-,48,16> 0.0 ("y"), s=w626, f=fxp<+/-,48,16> 0.00030517578125 ("y")) -> (s? t:f=w632:fxp<+/-,48,16>)
                                n164 = xnode "High Throughput Divide"("x"=w644, "y"=w641) -> ("x/y"=w643:fxp<+/-,48,16>)
                                n165 = xnode "High Throughput Divide"("x"=w642, "y"=w641) -> ("x/y"=w640:fxp<+/-,48,16>)
                                n166 = xnode ("High Throughput Add")("x"=w632, "y"=w656) -> ("x+y"=w646:fxp<+/-,48,16>)
                                n167 = xnode "High Throughput Subtract"("x"=w659, "y"=w640) -> ("x-y"=w658:fxp<+/-,48,16>)
                                n168 = Absolute Value(x=w658) -> (abs(x)=w637:fxp<+,48,16>)
                                n169 = Less Or Equal?(x=w646, y=fxp<+/-,48,16> 9.75) -> (x <= y?=w648:bool)
                                n170 = Greater Or Equal?(x=w646, y=fxp<+/-,48,16> -0.125) -> (x >= y?=w649:bool)
                                n171 = And(x=w649, y=w648) -> (x .and. y?=w647:bool)
                                n172 = Less Or Equal?(x=w637, y=w636) -> (x <= y?=w638:bool)
                                n173 = xnode ("Register Read")() -> ("Data"=w652:bool)  [unwired: 1 in, 1 out]
                                n174 = Not(x=w638) -> (.not. x?=w645:bool)
                                n175 = Compound Arithmetic op=AND(w638, invert w652, w647) -> (w622:bool)
                                n176 = Not(x=w622) -> (.not. x?=w635:bool)
                                n177 = Select(t=w646, s=w622, f=w656) -> (s? t:f=w655:fxp<+/-,48,16>)
                                }
                                frame #2 {
                                n178 = xnode "FPGA I/O Node"("Connector0/AO2"=w729) -> ()  [unwired: 1 in, 1 out]
                                }
                                frame #3 {
                                n179 = Not(x=w734) -> (.not. x?=w733:bool)
                                n180 = Less?(x=w732, y=8099 ("f")) -> (x < y?=w730:bool)
                                n181 = case shown="True" w733 {
                                tunnel: w740 -> [_ w753]
                                tunnel: w732 -> [_ w749]
                                tunnel: w743 -> [_ w747]
                                tunnel: w742 -> [_ w746]
                                frame False {
                                }
                                frame True {
                                n182 = Add(x=w749, y=8) -> (x+y=w751:i32)
                                n183 = Add(x=w749, y=8108) -> (x+y=w748:i32)
                                n184 = case shown="2" w753 {
                                tunnel: w751 -> [w757 w781 w809]
                                tunnel: w748 -> [w756 w780 w808]
                                tunnel: w747 -> [w755 w782 w807]
                                tunnel: w746 -> [w754 w783 w806]
                                frame 0, Default {
                                n185 = stacked-sequence {
                                tunnel: w757 -> [w761 _]
                                tunnel: w756 -> [_ w772]
                                tunnel: w755 -> [w760 _]
                                tunnel: w754 -> [_ w771]
                                frame #0 {
                                n186 = node-c288() -> (w759:T1)  [unwired: 1 in]
                                n187 = timed-loop {
                                timing: w759 -> [_]
                                timing-out: [_] -> w758
                                tunnel: w761 -> [w764]
                                tunnel: w760 -> [w763]
                                stop <- TRUE stop-if-true
                                n188 = xnode ("Memory Method Node")("Address"=w764, "Data"=w763) -> ()  [unwired: 1 in, 1 out]
                                }
                                n189 = node-c288(w758) -> ()
                                }
                                frame #1 {
                                n190 = node-c288() -> (w770:T1)  [unwired: 1 in]
                                n191 = timed-loop {
                                timing: w770 -> [_]
                                timing-out: [_] -> w769
                                tunnel: w772 -> [w775]
                                tunnel: w771 -> [w774]
                                stop <- TRUE stop-if-true
                                n192 = xnode ("Memory Method Node")("Address"=w775, "Data"=w774) -> ()  [unwired: 1 in, 1 out]
                                }
                                n193 = node-c288(w769) -> ()
                                }
                                }
                                }
                                frame 1 {
                                n194 = stacked-sequence {
                                tunnel: w783 -> [_ w798]
                                tunnel: w782 -> [w787 _]
                                tunnel: w781 -> [w786 _]
                                tunnel: w780 -> [_ w797]
                                frame #0 {
                                n195 = node-c288() -> (w785:T1)  [unwired: 1 in]
                                n196 = timed-loop {
                                timing: w785 -> [_]
                                timing-out: [_] -> w784
                                tunnel: w787 -> [w790]
                                tunnel: w786 -> [w789]
                                stop <- TRUE stop-if-true
                                n197 = xnode ("Memory Method Node")("Address"=w789, "Data"=w790) -> ()  [unwired: 1 in, 1 out]
                                }
                                n198 = node-c288(w784) -> ()
                                }
                                frame #1 {
                                n199 = node-c288() -> (w796:T1)  [unwired: 1 in]
                                n200 = timed-loop {
                                timing: w796 -> [_]
                                timing-out: [_] -> w795
                                tunnel: w798 -> [w801]
                                tunnel: w797 -> [w800]
                                stop <- TRUE stop-if-true
                                n201 = xnode ("Memory Method Node")("Address"=w800, "Data"=w801) -> ()  [unwired: 1 in, 1 out]
                                }
                                n202 = node-c288(w795) -> ()
                                }
                                }
                                }
                                frame 2 {
                                n203 = stacked-sequence {
                                tunnel: w806 -> [_ w824]
                                tunnel: w807 -> [w813 _]
                                tunnel: w809 -> [w812 _]
                                tunnel: w808 -> [_ w823]
                                frame #0 {
                                n204 = node-c288() -> (w811:T1)  [unwired: 1 in]
                                n205 = timed-loop {
                                timing: w811 -> [_]
                                timing-out: [_] -> w810
                                tunnel: w813 -> [w814]
                                tunnel: w812 -> [w815]
                                stop <- TRUE stop-if-true
                                n206 = xnode ("Memory Method Node")("Address"=w815, "Data"=w814) -> ()  [unwired: 1 in, 1 out]
                                }
                                n207 = node-c288(w810) -> ()
                                }
                                frame #1 {
                                n208 = node-c288() -> (w822:T1)  [unwired: 1 in]
                                n209 = timed-loop {
                                timing: w822 -> [_]
                                timing-out: [_] -> w821
                                tunnel: w824 -> [w825]
                                tunnel: w823 -> [w826]
                                stop <- TRUE stop-if-true
                                n210 = xnode ("Memory Method Node")("Address"=w826, "Data"=w825) -> ()  [unwired: 1 in, 1 out]
                                }
                                n211 = node-c288(w821) -> ()
                                }
                                }
                                }
                                }
                                }
                                }
                                n212 = Increment(x=w732) -> (x+1=w745:i32)
                                n213 = Select(t=w745, s=w730, f=0) -> (s? t:f=w744:i32)
                                }
                                frame #4 {
                                n214 = call "Tick Count2"() -> ("Tick Count(uSec)"=w840:u32)
                                n215 = local read "AppRate_NF us"() -> (w832:i32)
                                n216 = Subtract(x=w840, y=w839) -> (x-y=w838:i32)
                                n217 = Subtract(x=w832, y=w838) -> (x-y=w837:i32)
                                n218 = In Range and Coerce(upper limit=80000, x=w837, lower limit=1) -> (coerced(x)=w834:i32)  [unwired: 1 out]
                                n219 = call "Wait9"("Count(uSec)"=w834) -> ()  [unwired: 1 out]
                                }
                              }
                            }
                          }
                          frame #5 {
                            n220 = xnode ("Register Read")() -> ("Data"=w850:bool)  [unwired: 1 in, 1 out]
                            n221 = Compound Arithmetic op=AND(w854, invert w850) -> (w857:bool)
                            n222 = case shown="True" w857 {
                              tunnel: w856 -> [_ w878]
                              tunnel: w855 -> [_ w879]
                              tunnel: w853 -> [w859 w877]
                              tunnel: [w859 w876] -> w852
                              tunnel: [FALSE w872] -> w849
                              tunnel: w847 -> [_ w871]
                              tunnel: w846 -> [_ w860]
                              frame False {
                              }
                              frame True {
                                w880 = fxp<+/-,48,16> 0.0 ("ZPeizoOffset")
                                n223 = for {
                                N: 16 -> [_]
                                shift-right: [w1198] -> w869
                                shift-left: w880 -> [w1202]
                                shift-right: [w1197] -> w866
                                shift-left: w880 -> [w1200]
                                shift-right: [w1194] -> w863
                                shift-left: w880 -> [w1196]
                                n224 = xnode "FPGA I/O Node"() -> ("Connector0/AI0"=w1201:fxp<+/-,27,5>, "Connector0/AI1"=w1199:fxp<+/-,27,5>, "Connector0/AI2"=w1195:fxp<+/-,27,5>)  [unwired: 3 in, 3 out]
                                n225 = xnode ("High Throughput Add")("x"=w1201, "y"=w1202) -> ("x+y"=w1198:fxp<+/-,48,16>)
                                n226 = xnode ("High Throughput Add")("x"=w1196, "y"=w1195) -> ("x+y"=w1194:fxp<+/-,48,16>)
                                n227 = xnode ("High Throughput Add")("x"=w1199, "y"=w1200) -> ("x+y"=w1197:fxp<+/-,48,16>)
                                }
                                n228 = feedback #1(u32 0 ("Timeout")) -> (w874:u32)
                                n229 = Increment(x=w874) -> (x+1=w861:u32)
                                "point_scanned" <- w861
                                n230 = feedback-in #1(w861) -> ()
                                n231 = local read "TotalPoints"() -> (w873:u32)
                                n232 = Greater Or Equal?(x=w861, y=w873) -> (x >= y?=w872:bool)
                                n233 = xnode "High Throughput Divide"("x"=w866, "y"=fxp<+/-,48,16> 16.0 ("ZPeizoOffset")) -> ("x/y"=w865:fxp<+/-,48,16>)
                                n234 = xnode "High Throughput Divide"("x"=w869, "y"=fxp<+/-,48,16> 16.0 ("ZPeizoOffset")) -> ("x/y"=w868:fxp<+/-,48,16>)
                                n235 = xnode "High Throughput Divide"("x"=w863, "y"=fxp<+/-,48,16> 16.0 ("ZPeizoOffset")) -> ("x/y"=w862:fxp<+/-,48,16>)
                                n236 = stacked-sequence {
                                tunnel: w868 -> [w963 _ _ _ _ _ _ _]
                                tunnel: w865 -> [_ w995 _ _ _ _ _ _]
                                tunnel: w862 -> [_ _ _ _ _ w1123 _ _]
                                tunnel: w879 -> [_ _ w1028 _ _ _ _ _]
                                tunnel: w878 -> [_ _ _ w1060 _ _ _ _]
                                tunnel: w877 -> [w964 w996 w1027 w1059 w1091 w1124 w1156 w1191]
                                tunnel: [_ _ _ _ _ _ _ w1189] -> w876
                                tunnel: w871 -> [_ _ _ _ _ _ w1155 _]
                                tunnel: w860 -> [_ _ _ _ w1092 _ _ _]
                                frame #0 {
                                n237 = case shown="0, Default" w964 {
                                tunnel: w963 -> [w967 w977 w985]
                                frame 0, Default {
                                n238 = node-c288() -> (w966:T1)  [unwired: 1 in]
                                n239 = timed-loop {
                                timing: w966 -> [_]
                                timing-out: [_] -> w965
                                tunnel: w967 -> [w969]
                                stop <- TRUE stop-if-true
                                n240 = xnode ("Memory Method Node")("Address"=u32 0, "Data"=w969) -> ()  [unwired: 1 in, 1 out]
                                }
                                n241 = node-c288(w965) -> ()
                                }
                                frame 1 {
                                n242 = node-c288() -> (w976:T1)  [unwired: 1 in]
                                n243 = timed-loop {
                                timing: w976 -> [_]
                                timing-out: [_] -> w975
                                tunnel: w977 -> [w979]
                                stop <- TRUE stop-if-true
                                n244 = xnode ("Memory Method Node")("Address"=u32 0, "Data"=w979) -> ()  [unwired: 1 in, 1 out]
                                }
                                n245 = node-c288(w975) -> ()
                                }
                                frame 2 {
                                n246 = node-c288() -> (w987:T1)  [unwired: 1 in]
                                n247 = timed-loop {
                                timing: w987 -> [_]
                                timing-out: [_] -> w986
                                tunnel: w985 -> [w988]
                                stop <- TRUE stop-if-true
                                n248 = xnode ("Memory Method Node")("Address"=u32 0, "Data"=w988) -> ()  [unwired: 1 in, 1 out]
                                }
                                n249 = node-c288(w986) -> ()
                                }
                                }
                                }
                                frame #1 {
                                n250 = case shown="2" w996 {
                                tunnel: w995 -> [w999 w1009 w1017]
                                frame 0, Default {
                                n251 = node-c288() -> (w998:T1)  [unwired: 1 in]
                                n252 = timed-loop {
                                timing: w998 -> [_]
                                timing-out: [_] -> w997
                                tunnel: w999 -> [w1001]
                                stop <- TRUE stop-if-true
                                n253 = xnode ("Memory Method Node")("Address"=u32 1, "Data"=w1001) -> ()  [unwired: 1 in, 1 out]
                                }
                                n254 = node-c288(w997) -> ()
                                }
                                frame 1 {
                                n255 = node-c288() -> (w1008:T1)  [unwired: 1 in]
                                n256 = timed-loop {
                                timing: w1008 -> [_]
                                timing-out: [_] -> w1007
                                tunnel: w1009 -> [w1011]
                                stop <- TRUE stop-if-true
                                n257 = xnode ("Memory Method Node")("Address"=u32 1, "Data"=w1011) -> ()  [unwired: 1 in, 1 out]
                                }
                                n258 = node-c288(w1007) -> ()
                                }
                                frame 2 {
                                n259 = node-c288() -> (w1019:T1)  [unwired: 1 in]
                                n260 = timed-loop {
                                timing: w1019 -> [_]
                                timing-out: [_] -> w1018
                                tunnel: w1017 -> [w1020]
                                stop <- TRUE stop-if-true
                                n261 = xnode ("Memory Method Node")("Address"=u32 1, "Data"=w1020) -> ()  [unwired: 1 in, 1 out]
                                }
                                n262 = node-c288(w1018) -> ()
                                }
                                }
                                }
                                frame #2 {
                                n263 = case shown="2" w1027 {
                                tunnel: w1028 -> [w1031 w1041 w1049]
                                frame 0, Default {
                                n264 = node-c288() -> (w1030:T1)  [unwired: 1 in]
                                n265 = timed-loop {
                                timing: w1030 -> [_]
                                timing-out: [_] -> w1029
                                tunnel: w1031 -> [w1033]
                                stop <- TRUE stop-if-true
                                n266 = xnode ("Memory Method Node")("Address"=u32 2, "Data"=w1033) -> ()  [unwired: 1 in, 1 out]
                                }
                                n267 = node-c288(w1029) -> ()
                                }
                                frame 1 {
                                n268 = node-c288() -> (w1040:T1)  [unwired: 1 in]
                                n269 = timed-loop {
                                timing: w1040 -> [_]
                                timing-out: [_] -> w1039
                                tunnel: w1041 -> [w1043]
                                stop <- TRUE stop-if-true
                                n270 = xnode ("Memory Method Node")("Address"=u32 2, "Data"=w1043) -> ()  [unwired: 1 in, 1 out]
                                }
                                n271 = node-c288(w1039) -> ()
                                }
                                frame 2 {
                                n272 = node-c288() -> (w1051:T1)  [unwired: 1 in]
                                n273 = timed-loop {
                                timing: w1051 -> [_]
                                timing-out: [_] -> w1050
                                tunnel: w1049 -> [w1052]
                                stop <- TRUE stop-if-true
                                n274 = xnode ("Memory Method Node")("Address"=u32 2, "Data"=w1052) -> ()  [unwired: 1 in, 1 out]
                                }
                                n275 = node-c288(w1050) -> ()
                                }
                                }
                                }
                                frame #3 {
                                n276 = case shown="2" w1059 {
                                tunnel: w1060 -> [w1063 w1073 w1081]
                                frame 0, Default {
                                n277 = node-c288() -> (w1062:T1)  [unwired: 1 in]
                                n278 = timed-loop {
                                timing: w1062 -> [_]
                                timing-out: [_] -> w1061
                                tunnel: w1063 -> [w1065]
                                stop <- TRUE stop-if-true
                                n279 = xnode ("Memory Method Node")("Address"=u32 3, "Data"=w1065) -> ()  [unwired: 1 in, 1 out]
                                }
                                n280 = node-c288(w1061) -> ()
                                }
                                frame 1 {
                                n281 = node-c288() -> (w1072:T1)  [unwired: 1 in]
                                n282 = timed-loop {
                                timing: w1072 -> [_]
                                timing-out: [_] -> w1071
                                tunnel: w1073 -> [w1075]
                                stop <- TRUE stop-if-true
                                n283 = xnode ("Memory Method Node")("Address"=u32 3, "Data"=w1075) -> ()  [unwired: 1 in, 1 out]
                                }
                                n284 = node-c288(w1071) -> ()
                                }
                                frame 2 {
                                n285 = node-c288() -> (w1083:T1)  [unwired: 1 in]
                                n286 = timed-loop {
                                timing: w1083 -> [_]
                                timing-out: [_] -> w1082
                                tunnel: w1081 -> [w1084]
                                stop <- TRUE stop-if-true
                                n287 = xnode ("Memory Method Node")("Address"=u32 3, "Data"=w1084) -> ()  [unwired: 1 in, 1 out]
                                }
                                n288 = node-c288(w1082) -> ()
                                }
                                }
                                }
                                frame #4 {
                                n289 = case shown="0, Default" w1091 {
                                tunnel: w1092 -> [w1095 w1105 w1113]
                                frame 0, Default {
                                n290 = node-c288() -> (w1094:T1)  [unwired: 1 in]
                                n291 = timed-loop {
                                timing: w1094 -> [_]
                                timing-out: [_] -> w1093
                                tunnel: w1095 -> [w1097]
                                stop <- TRUE stop-if-true
                                n292 = xnode ("Memory Method Node")("Address"=u32 4, "Data"=w1097) -> ()  [unwired: 1 in, 1 out]
                                }
                                n293 = node-c288(w1093) -> ()
                                }
                                frame 1 {
                                n294 = node-c288() -> (w1104:T1)  [unwired: 1 in]
                                n295 = timed-loop {
                                timing: w1104 -> [_]
                                timing-out: [_] -> w1103
                                tunnel: w1105 -> [w1107]
                                stop <- TRUE stop-if-true
                                n296 = xnode ("Memory Method Node")("Address"=u32 4, "Data"=w1107) -> ()  [unwired: 1 in, 1 out]
                                }
                                n297 = node-c288(w1103) -> ()
                                }
                                frame 2 {
                                n298 = node-c288() -> (w1115:T1)  [unwired: 1 in]
                                n299 = timed-loop {
                                timing: w1115 -> [_]
                                timing-out: [_] -> w1114
                                tunnel: w1113 -> [w1116]
                                stop <- TRUE stop-if-true
                                n300 = xnode ("Memory Method Node")("Address"=u32 4, "Data"=w1116) -> ()  [unwired: 1 in, 1 out]
                                }
                                n301 = node-c288(w1114) -> ()
                                }
                                }
                                }
                                frame #5 {
                                n302 = case shown="2" w1124 {
                                tunnel: w1123 -> [w1127 w1137 w1145]
                                frame 0, Default {
                                n303 = node-c288() -> (w1126:T1)  [unwired: 1 in]
                                n304 = timed-loop {
                                timing: w1126 -> [_]
                                timing-out: [_] -> w1125
                                tunnel: w1127 -> [w1129]
                                stop <- TRUE stop-if-true
                                n305 = xnode ("Memory Method Node")("Address"=u32 5, "Data"=w1129) -> ()  [unwired: 1 in, 1 out]
                                }
                                n306 = node-c288(w1125) -> ()
                                }
                                frame 1 {
                                n307 = node-c288() -> (w1136:T1)  [unwired: 1 in]
                                n308 = timed-loop {
                                timing: w1136 -> [_]
                                timing-out: [_] -> w1135
                                tunnel: w1137 -> [w1139]
                                stop <- TRUE stop-if-true
                                n309 = xnode ("Memory Method Node")("Address"=u32 5, "Data"=w1139) -> ()  [unwired: 1 in, 1 out]
                                }
                                n310 = node-c288(w1135) -> ()
                                }
                                frame 2 {
                                n311 = node-c288() -> (w1147:T1)  [unwired: 1 in]
                                n312 = timed-loop {
                                timing: w1147 -> [_]
                                timing-out: [_] -> w1146
                                tunnel: w1145 -> [w1148]
                                stop <- TRUE stop-if-true
                                n313 = xnode ("Memory Method Node")("Address"=u32 5, "Data"=w1148) -> ()  [unwired: 1 in, 1 out]
                                }
                                n314 = node-c288(w1146) -> ()
                                }
                                }
                                }
                                frame #6 {
                                n315 = case shown="2" w1156 {
                                tunnel: w1155 -> [w1159 w1169 w1177]
                                frame 0, Default {
                                n316 = node-c288() -> (w1158:T1)  [unwired: 1 in]
                                n317 = timed-loop {
                                timing: w1158 -> [_]
                                timing-out: [_] -> w1157
                                tunnel: w1159 -> [w1161]
                                stop <- TRUE stop-if-true
                                n318 = xnode ("Memory Method Node")("Address"=u32 6, "Data"=w1161) -> ()  [unwired: 1 in, 1 out]
                                }
                                n319 = node-c288(w1157) -> ()
                                }
                                frame 1 {
                                n320 = node-c288() -> (w1168:T1)  [unwired: 1 in]
                                n321 = timed-loop {
                                timing: w1168 -> [_]
                                timing-out: [_] -> w1167
                                tunnel: w1169 -> [w1171]
                                stop <- TRUE stop-if-true
                                n322 = xnode ("Memory Method Node")("Address"=u32 6, "Data"=w1171) -> ()  [unwired: 1 in, 1 out]
                                }
                                n323 = node-c288(w1167) -> ()
                                }
                                frame 2 {
                                n324 = node-c288() -> (w1179:T1)  [unwired: 1 in]
                                n325 = timed-loop {
                                timing: w1179 -> [_]
                                timing-out: [_] -> w1178
                                tunnel: w1177 -> [w1180]
                                stop <- TRUE stop-if-true
                                n326 = xnode ("Memory Method Node")("Address"=u32 6, "Data"=w1180) -> ()  [unwired: 1 in, 1 out]
                                }
                                n327 = node-c288(w1178) -> ()
                                }
                                }
                                }
                                frame #7 {
                                n328 = xnode ("FIFO Method Node")("Element"=w1191, "Timeout"=0) -> ()  [unwired: 1 in, 2 out]
                                n329 = Increment(x=w1191) -> (x+1=w1190:u8)
                                n330 = Greater Or Equal?(x=w1190, y=u8 3) -> (x >= y?=w1192:bool)
                                n331 = Select(t=w1191, s=w1192, f=u8 0) -> (s? t:f=w1189:u8)
                                }
                                }
                              }
                            }
                            n332 = Or(x=w850, y=w849) -> (x .or. y?=w848:bool)
                          }
                          frame #6 {
                            n333 = xnode ("Register Read")() -> ("Data"=w1206:bool)  [unwired: 1 in, 1 out]
                            n334 = Less Or Equal To 0?(x=w1207) -> (x <= 0?=w1205:bool)
                            n335 = Or(x=w1206, y=w1205) -> (x .or. y?=w1204:bool)
                            n336 = case shown="False" w1204 {
                              tunnel: w1207 -> [w1214 w1228]
                              tunnel: [w1216 w1228] -> w1209
                              tunnel: fxp<+/-,48,16> 0.00030517578125 ("y") -> [w1215 _]
                              tunnel: w1208 -> [w1212 _]
                              frame False {
                                n337 = xnode "High Throughput Subtract"("x"=w1214, "y"=w1212) -> ("x-y"=w1213:fxp<+/-,48,16>)
                                n338 = while {
                                shift-right: [w1221] -> w1216
                                shift-left: w1214 -> [w1227]
                                tunnel: w1215 -> [w1220]
                                tunnel: w1213 -> [w1219]
                                stop <- w1222 stop-if-true
                                n339 = xnode "High Throughput Subtract"("x"=w1227, "y"=w1220) -> ("x-y"=w1223:fxp<+/-,48,16>)
                                n340 = xnode ("Register Read")() -> ("Data"=w1226:bool)  [unwired: 1 in, 1 out]
                                n341 = Less Or Equal To 0?(x=w1223) -> (x <= 0?=w1224:bool)
                                n342 = Less Or Equal?(x=w1223, y=w1219) -> (x <= y?=w1225:bool)
                                n343 = Select(t=fxp<+/-,48,16> 0.0, s=w1224, f=w1223) -> (s? t:f=w1221:fxp<+/-,48,16>)
                                n344 = local read "RetRate us"() -> (w1217:i32)
                                n345 = xnode "FPGA I/O Node"("Connector0/AO2"=w1221) -> ()  [unwired: 1 in, 1 out]
                                n346 = Compound Arithmetic op=OR(w1224, w1225, w1226) -> (w1222:bool)
                                n347 = call "Wait11"("Count(uSec)"=w1217) -> ()  [unwired: 1 out]
                                }
                              }
                              frame True {
                              }
                            }
                          }
                          frame #7 {
                            n348 = call "Wait21"("Count(mSec)"=u8 10) -> ()  [unwired: 1 out]
                          }
                        }
                      }
                      frame True {
                        n349 = xnode ("Register Read")() -> ("Data"=w1233:bool)  [unwired: 1 in, 1 out]
                        n350 = Not(x=w1236) -> (.not. x?=w1235:bool)
                        n351 = Or(x=w1235, y=w1233) -> (x .or. y?=w1234:bool)
                      }
                    }
                  }
                }
              }
            }
            frame True {
            }
          }
        }
        frame #4 {
          n352 = while {
            shift-right: [w1247] -> _
            shift-left: w1243 -> [w1252]
            tunnel: fxp<+/-,48,16> 0.00030517578125 ("y") -> [w1246]
            stop <- w1248 stop-if-true
            w1244 = fxp<+/-,48,16> 0.0 ("t")
            n353 = xnode "High Throughput Subtract"("x"=w1252, "y"=w1246) -> ("x-y"=w1249:fxp<+/-,48,16>)
            n354 = Less Or Equal To 0?(x=w1249) -> (x <= 0?=w1250:bool)
            n355 = Less Or Equal?(x=w1249, y=w1244) -> (x <= y?=w1251:bool)
            n356 = Select(t=w1244, s=w1250, f=w1249) -> (s? t:f=w1247:fxp<+/-,48,16>)
            n357 = local read "RetRate us"() -> (w1245:i32)
            n358 = xnode "FPGA I/O Node"("Connector0/AO2"=w1247) -> ()  [unwired: 1 in, 1 out]
            n359 = Compound Arithmetic op=OR(w1250, w1251) -> (w1248:bool)
            n360 = call "Wait12"("Count(uSec)"=w1245) -> ()  [unwired: 1 out]
          }
          n361 = xnode "FPGA I/O Node"() -> ("Connector0/AI0"=w1242:fxp<+/-,27,5>, "Connector0/AI1"=w1241:fxp<+/-,27,5>)  [unwired: 2 in, 2 out]
        }
        frame #5 {
          n362 = call "Wait15"("Count(uSec)"=u8 100) -> ()  [unwired: 1 out]
        }
        frame #6 {
          n363 = xnode ("Register Read")() -> ("Data"=w1256:bool)  [unwired: 1 in, 1 out]
          n364 = local read "LastScan"() -> (w1258:bool)
          n365 = Or(x=w1256, y=w1258) -> (x .or. y?=w1257:bool)
          n366 = case shown="True" w1257 {
            tunnel: w1260 -> [_ w1264]
            tunnel: w1259 -> [_ w1261]
            frame False {
            }
            frame True {
              n367 = while {
                shift-right: [w1268] -> _
                shift-left: w1261 -> [w1273]
                tunnel: fxp<+/-,48,16> 0.0048828125 ("y") -> [w1267]
                stop <- w1269 stop-if-true
                w1266 = fxp<+/-,48,16> 0.0 ("t")
                n368 = xnode "High Throughput Subtract"("x"=w1273, "y"=w1267) -> ("x-y"=w1270:fxp<+/-,48,16>)
                n369 = Less Or Equal To 0?(x=w1270) -> (x <= 0?=w1271:bool)
                n370 = Less Or Equal?(x=w1270, y=w1266) -> (x <= y?=w1272:bool)
                n371 = Select(t=w1266, s=w1271, f=w1270) -> (s? t:f=w1268:fxp<+/-,48,16>)
                n372 = xnode "FPGA I/O Node"("Connector0/AO1"=w1268) -> ()  [unwired: 1 in, 1 out]
                n373 = Compound Arithmetic op=OR(w1271, w1272) -> (w1269:bool)
                n374 = call "Wait14"("Count(uSec)"=u16 100) -> ()  [unwired: 1 out]
              }
              n375 = while {
                shift-right: [w1277] -> _
                shift-left: w1264 -> [w1282]
                tunnel: fxp<+/-,48,16> 0.0048828125 ("y") -> [w1276]
                stop <- w1278 stop-if-true
                w1275 = fxp<+/-,48,16> 0.0 ("t")
                n376 = xnode "High Throughput Subtract"("x"=w1282, "y"=w1276) -> ("x-y"=w1279:fxp<+/-,48,16>)
                n377 = Less Or Equal To 0?(x=w1279) -> (x <= 0?=w1280:bool)
                n378 = Less Or Equal?(x=w1279, y=w1275) -> (x <= y?=w1281:bool)
                n379 = Select(t=w1275, s=w1280, f=w1279) -> (s? t:f=w1277:fxp<+/-,48,16>)
                n380 = xnode "FPGA I/O Node"("Connector0/AO0"=w1277) -> ()  [unwired: 1 in, 1 out]
                n381 = Compound Arithmetic op=OR(w1280, w1281) -> (w1278:bool)
                n382 = call "Wait13"("Count(uSec)"=u16 100) -> ()  [unwired: 1 out]
              }
            }
          }
        }
        frame #7 {
          n383 = call "Wait16"("Count(uSec)"=u8 100) -> ()  [unwired: 1 out]
        }
        frame #8 {
          n384 = local write "ScanFinished?"(TRUE ("ScanFinished?")) -> ()
        }
      }
      n385 = while {
        stop <- w37 stop-if-true
        n386 = xnode ("Register Read")() -> ("Data"=w38:bool)  [unwired: 1 in, 1 out]
        n387 = xnode ("FIFO Method Node")() -> ("Number of Elements to Read"=w36:u32)  [unwired: 1 in, 1 out]
        n388 = local read "ScanFinished?"() -> (w39:bool)
        n389 = call "Wait8"("Count(uSec)"=u8 200 ("Count(mSec)")) -> ()  [unwired: 1 out]
        n390 = Or(x=w39, y=w38) -> (x .or. y?=w37:bool)
        n391 = Greater Than 0?(x=w36) -> (x > 0?=w35:bool)
        n392 = case shown="True" w35 {
          frame False {
          }
          frame True {
            # "push data in swapbuffer from target to host and clear buffer synchronously"
            n393 = flat-sequence {
              frame #0 {
              }
              frame #1 {
                n394 = xnode ("FIFO Method Node")("Timeout"=8192) -> ("Element"=w41:u8)  [unwired: 1 in, 2 out]
                n395 = case shown="0, Default" w41 {
                  frame 0, Default {
                    n396 = flat-sequence {
                      frame #0 {
                        n397 = node-c288(refnum<k21> "8MHz" ("Source Name")) -> (w45:T1)
                        n398 = timed-loop {
                          timing: w45 -> [_]
                          timing-out: [_] -> w44
                          shift-right: [w47] -> _
                          shift-left: _ -> [w54]
                          shift-right: [w54] -> _
                          shift-left: _ -> [w53]
                          shift-right: [w53] -> _
                          shift-left: _ -> [w50]
                          i -> [w46]
                          stop <- w51 stop-if-true
                          n399 = Greater Or Equal?(x=w46, y=16386) -> (x >= y?=w51:bool)
                          n400 = Greater Or Equal?(x=w46, y=3) -> (x >= y?=w49:bool)
                          n401 = case shown="True" w49 {
                            tunnel: w50 -> [_ w55]
                            frame False {
                            }
                            frame True {
                              n402 = xnode ("FIFO Method Node")("Element"=w55, "Timeout"=0) -> ()  [unwired: 1 in, 2 out]
                            }
                          }
                          n403 = xnode ("Memory Method Node")("Address"=w46) -> ("Data"=w47:fxp<+/-,48,16>)  [unwired: 1 in, 1 out]
                        }
                        n404 = node-c288(w44) -> ()
                      }
                      frame #1 {
                        n405 = node-c288() -> (w64:T1)  [unwired: 1 in]
                        n406 = timed-loop {
                          timing: w64 -> [_]
                          timing-out: [_] -> w63
                          i -> [w65]
                          stop <- w66 stop-if-true
                          n407 = xnode ("Memory Method Node")("Address"=w65, "Data"=fxp<+/-,48,16> -100.0) -> ()  [unwired: 1 in, 1 out]
                          n408 = Greater Or Equal?(x=w65, y=16383) -> (x >= y?=w66:bool)
                        }
                        n409 = node-c288(w63) -> ()
                      }
                    }
                  }
                  frame 1 {
                    n410 = flat-sequence {
                      frame #0 {
                        n411 = node-c288(refnum<k21> "8MHz" ("Source Name")) -> (w75:T1)
                        n412 = timed-loop {
                          timing: w75 -> [_]
                          timing-out: [_] -> w74
                          shift-right: [w84] -> _
                          shift-left: _ -> [w83]
                          shift-right: [w83] -> _
                          shift-left: _ -> [w82]
                          shift-right: [w82] -> _
                          shift-left: _ -> [w79]
                          i -> [w78]
                          stop <- w80 stop-if-true
                          n413 = Greater Or Equal?(x=w78, y=3) -> (x >= y?=w77:bool)
                          n414 = Greater Or Equal?(x=w78, y=16386) -> (x >= y?=w80:bool)
                          n415 = case shown="True" w77 {
                            tunnel: w79 -> [_ w85]
                            frame False {
                            }
                            frame True {
                              n416 = xnode ("FIFO Method Node")("Element"=w85, "Timeout"=0) -> ()  [unwired: 1 in, 2 out]
                            }
                          }
                          n417 = xnode ("Memory Method Node")("Address"=w78) -> ("Data"=w84:fxp<+/-,48,16>)  [unwired: 1 in, 1 out]
                        }
                        n418 = node-c288(w74) -> ()
                      }
                      frame #1 {
                        n419 = node-c288() -> (w94:T1)  [unwired: 1 in]
                        n420 = timed-loop {
                          timing: w94 -> [_]
                          timing-out: [_] -> w93
                          i -> [w95]
                          stop <- w97 stop-if-true
                          n421 = xnode ("Memory Method Node")("Address"=w95, "Data"=fxp<+/-,48,16> -100.0) -> ()  [unwired: 1 in, 1 out]
                          n422 = Greater Or Equal?(x=w95, y=16383) -> (x >= y?=w97:bool)
                        }
                        n423 = node-c288(w93) -> ()
                      }
                    }
                  }
                  frame 2 {
                    n424 = flat-sequence {
                      frame #0 {
                        n425 = node-c288(refnum<k21> "8MHz" ("Source Name")) -> (w105:T1)
                        n426 = timed-loop {
                          timing: w105 -> [_]
                          timing-out: [_] -> w104
                          shift-right: [w106] -> _
                          shift-left: _ -> [w114]
                          shift-right: [w114] -> _
                          shift-left: _ -> [w113]
                          shift-right: [w113] -> _
                          shift-left: _ -> [w110]
                          i -> [w107]
                          stop <- w111 stop-if-true
                          n427 = Greater Or Equal?(x=w107, y=3) -> (x >= y?=w109:bool)
                          n428 = Greater Or Equal?(x=w107, y=16386) -> (x >= y?=w111:bool)
                          n429 = case shown="True" w109 {
                            tunnel: w110 -> [_ w115]
                            frame False {
                            }
                            frame True {
                              n430 = xnode ("FIFO Method Node")("Element"=w115, "Timeout"=0) -> ()  [unwired: 1 in, 2 out]
                            }
                          }
                          n431 = xnode ("Memory Method Node")("Address"=w107) -> ("Data"=w106:fxp<+/-,48,16>)  [unwired: 1 in, 1 out]
                        }
                        n432 = node-c288(w104) -> ()
                      }
                      frame #1 {
                        n433 = node-c288() -> (w124:T1)  [unwired: 1 in]
                        n434 = timed-loop {
                          timing: w124 -> [_]
                          timing-out: [_] -> w123
                          i -> [w126]
                          stop <- w127 stop-if-true
                          n435 = xnode ("Memory Method Node")("Address"=w126, "Data"=fxp<+/-,48,16> -100.0) -> ()  [unwired: 1 in, 1 out]
                          n436 = Greater Or Equal?(x=w126, y=16383) -> (x >= y?=w127:bool)
                        }
                        n437 = node-c288(w123) -> ()
                      }
                    }
                  }
                }
              }
              frame #2 {
              }
            }
          }
        }
      }
    }
    frame #4 {
      n438 = local write "TargetDone?"(TRUE ("TargetDone?")) -> ()
    }
  }
